vi "configure.vi"(8 "error in (no error)":errorcluster, 9 "Value":i32, 10 "ILC":refnum<class "ILC.lvclass">, 11 "IConfigureILCStrategy in":refnum<class "ConfigureILCDAC3Strategy.lvclass">) -> (0 "error out":errorcluster, 2 "ILC 2":refnum<class "ILC.lvclass">, 3 "IConfigureILCStrategy out":refnum<class "ConfigureILCDAC3Strategy.lvclass">)   [LabVIEW 2016, in "ConfigureILCDAC3Strategy.lvclass"]
uses:
  ConfigureILCDAC3Strategy.lvclass
  Common_ILC/ILC/ILC.lvclass
  Common_ILC/ILC/ILC.lvclass/ILC.ctl
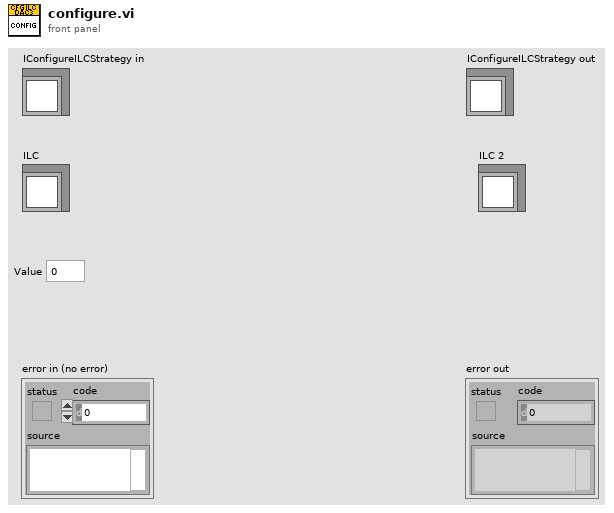
[diagram p1: front panel]
types:
  T1 = typedef "ILCCommon.lvlib/ILCTypedefs.lvlib/Outputs.ctl" = cluster{"Step & Direction":i16, "Blower RPM":u8, "PWM (SSR)":u8, "Ch1":u16, "Ch2":u16, "Ch3":u16, "Ch4":u16}
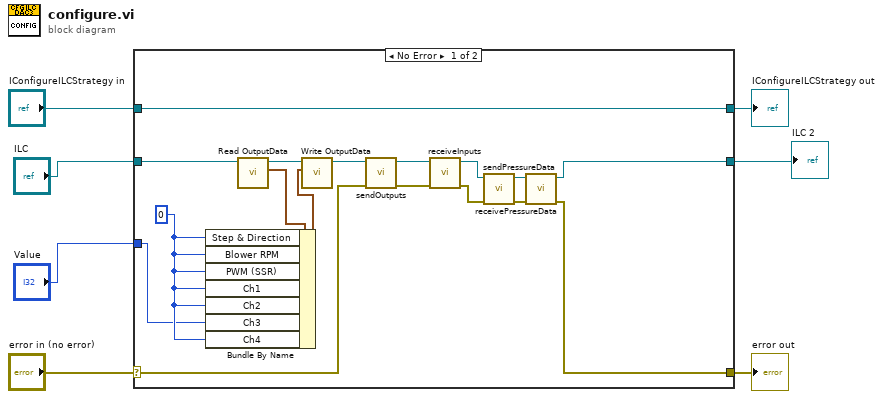
[diagram p0: block diagram]
diagram:
  n1 = case shown="No Error" "error in (no error)" {
    selector: "error in (no error)" -> [w19 w27]
    tunnel: [w10 w27] -> w6
    tunnel: [w24 w26] -> w4
    tunnel: "IConfigureILCStrategy in" -> [w24 w26]
    tunnel: "ILC" -> [w23 w25]
    tunnel: "Value" -> [w14 _]
    tunnel: [w8 w25] -> w1
    frame No Error {
      w17 = i16 0 ("Step & Direction")
      n2 = call "Read OutputData.vi"("ILC in"=w23) -> ("OutputData"=w16:T1, "ILC out"=w22:refnum<class "ILC.lvclass">)  [unwired: 9 in]
      n3 = Bundle By Name(cluster=w16, "Step & Direction"=w17, "Blower RPM"=w17, "PWM (SSR)"=w17, "Ch1"=w17, "Ch2"=w17, "Ch3"=w14, "Ch4"=w17) -> (w15:T1)
      n4 = call "Write OutputData.vi"("OutputData"=w15, "ILC in"=w22) -> ("ILC out"=w21:refnum<class "ILC.lvclass">)  [unwired: 9 in]
      n5 = call "sendOutputs.vi"("error in (no error)"=w19, "ILC in"=w21) -> ("error out"=w18:errorcluster, "ILC out"=w20:refnum<class "ILC.lvclass">)  [unwired: 8 in]
      n6 = call "receiveInputs.vi"("error in (no error)"=w18, "ILC in"=w20) -> ("error out"=w11:errorcluster, "ILC out"=w9:refnum<class "ILC.lvclass">)  [unwired: 6 in, 2 out]
      n7 = call "sendPressureData.vi"("error in (no error)"=w11, "ILC in"=w9) -> ("error out"=w13:errorcluster, "ILC out"=w12:refnum<class "ILC.lvclass">)  [unwired: 8 in]
      n8 = call "receivePressureData.vi"("error in (no error)"=w13, "ILC in"=w12) -> ("error out"=w10:errorcluster, "ILC out"=w8:refnum<class "ILC.lvclass">)  [unwired: 8 in]
    }
    frame Error {
    }
  }
  "error out" <- w6
  "IConfigureILCStrategy out" <- w4
  "ILC 2" <- w1
